vi "SCE_screen_main.vi"() -> ()   [LabVIEW 2018]
uses:
  SCE_VIC-II_registry.ctl
  SCE_character_bitmap.ctl
  CIA/CIA1/CIA1_glb.vi
panel:
  out "matrix":bool[][](array[boolean])
  out "VIC-II":T1
  out "Charset ROM":path=path "D:/work/experimets/C64/rom/characters.901225-01.bin"
  out "main time":u32
  out "Current State":string
  out "screen":picture
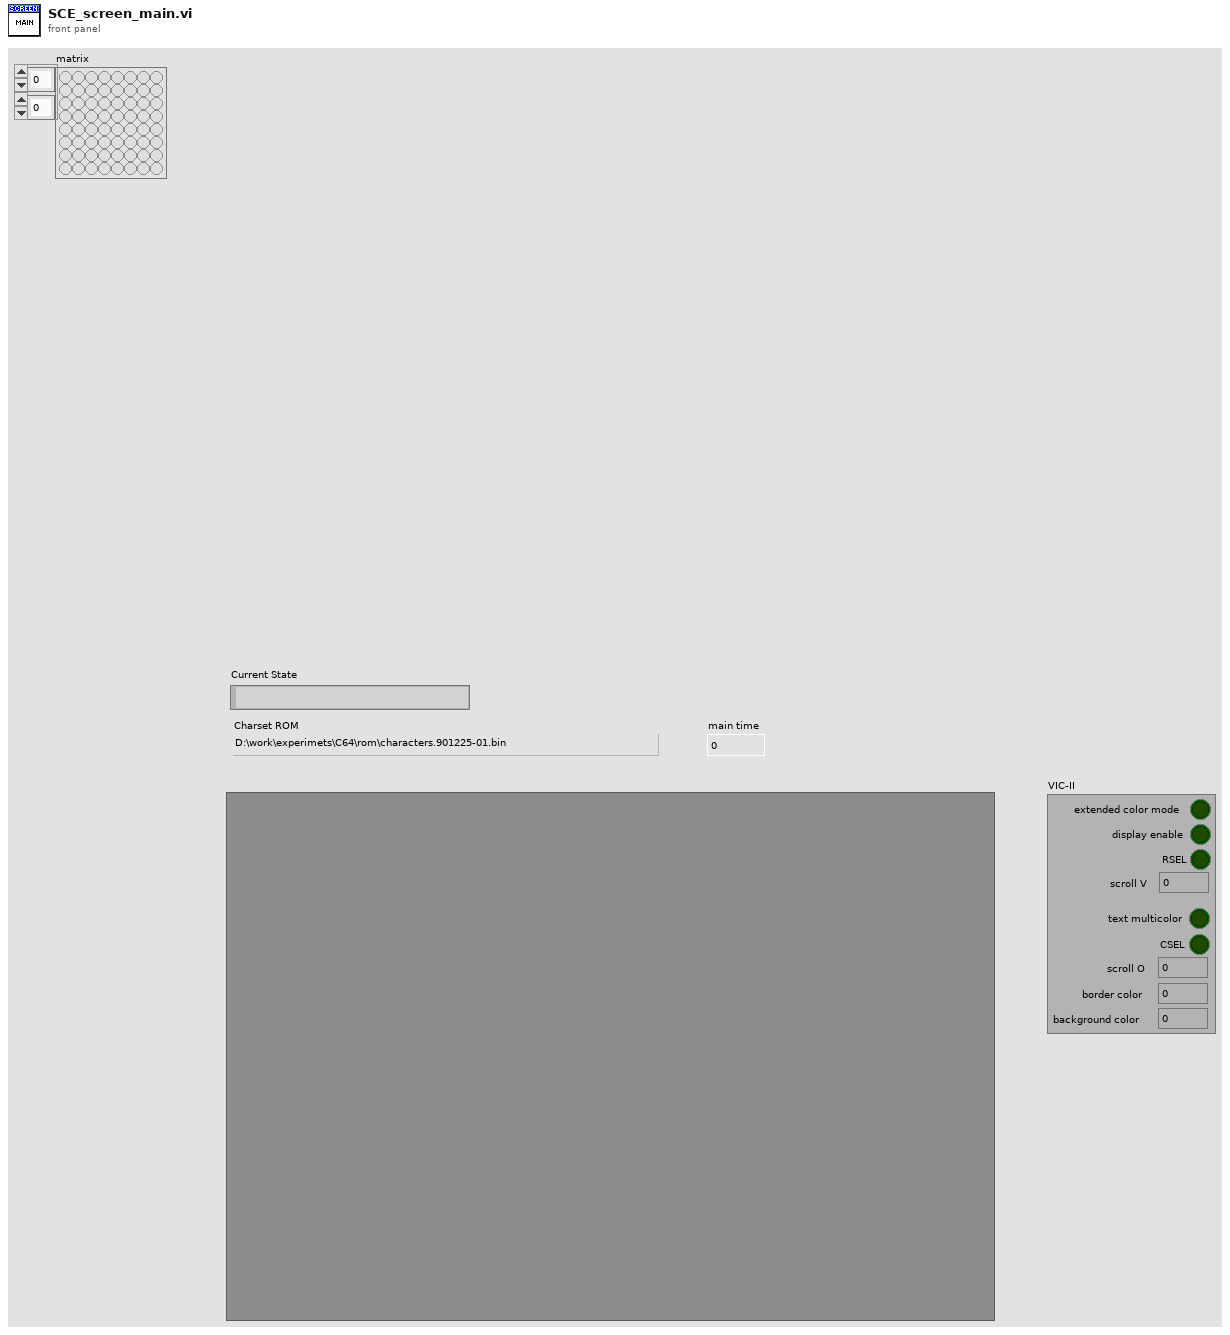
[diagram p1: front panel]
types:
  T1 = typedef "SCE_VIC-II_registry.ctl" = cluster{"extended color mode":bool, "display enable":bool, "RSEL":bool, "scroll V":u8, "text multicolor":bool, "CSEL":bool, "scroll O":u8, "border color":u8, "background color":u8}
  T2 = typedef "SCE_character_bitmap.ctl" = cluster{"ID":i32, "character bitmap":u8[][]}
  T3 = typedef "SCE_VIC-II_reg_D018.ctl" = cluster{"charset mode":enum16{"ROM set 1", "ROM set 2", "RAM"}, "charset addr":u16, "video ram addr":u16}
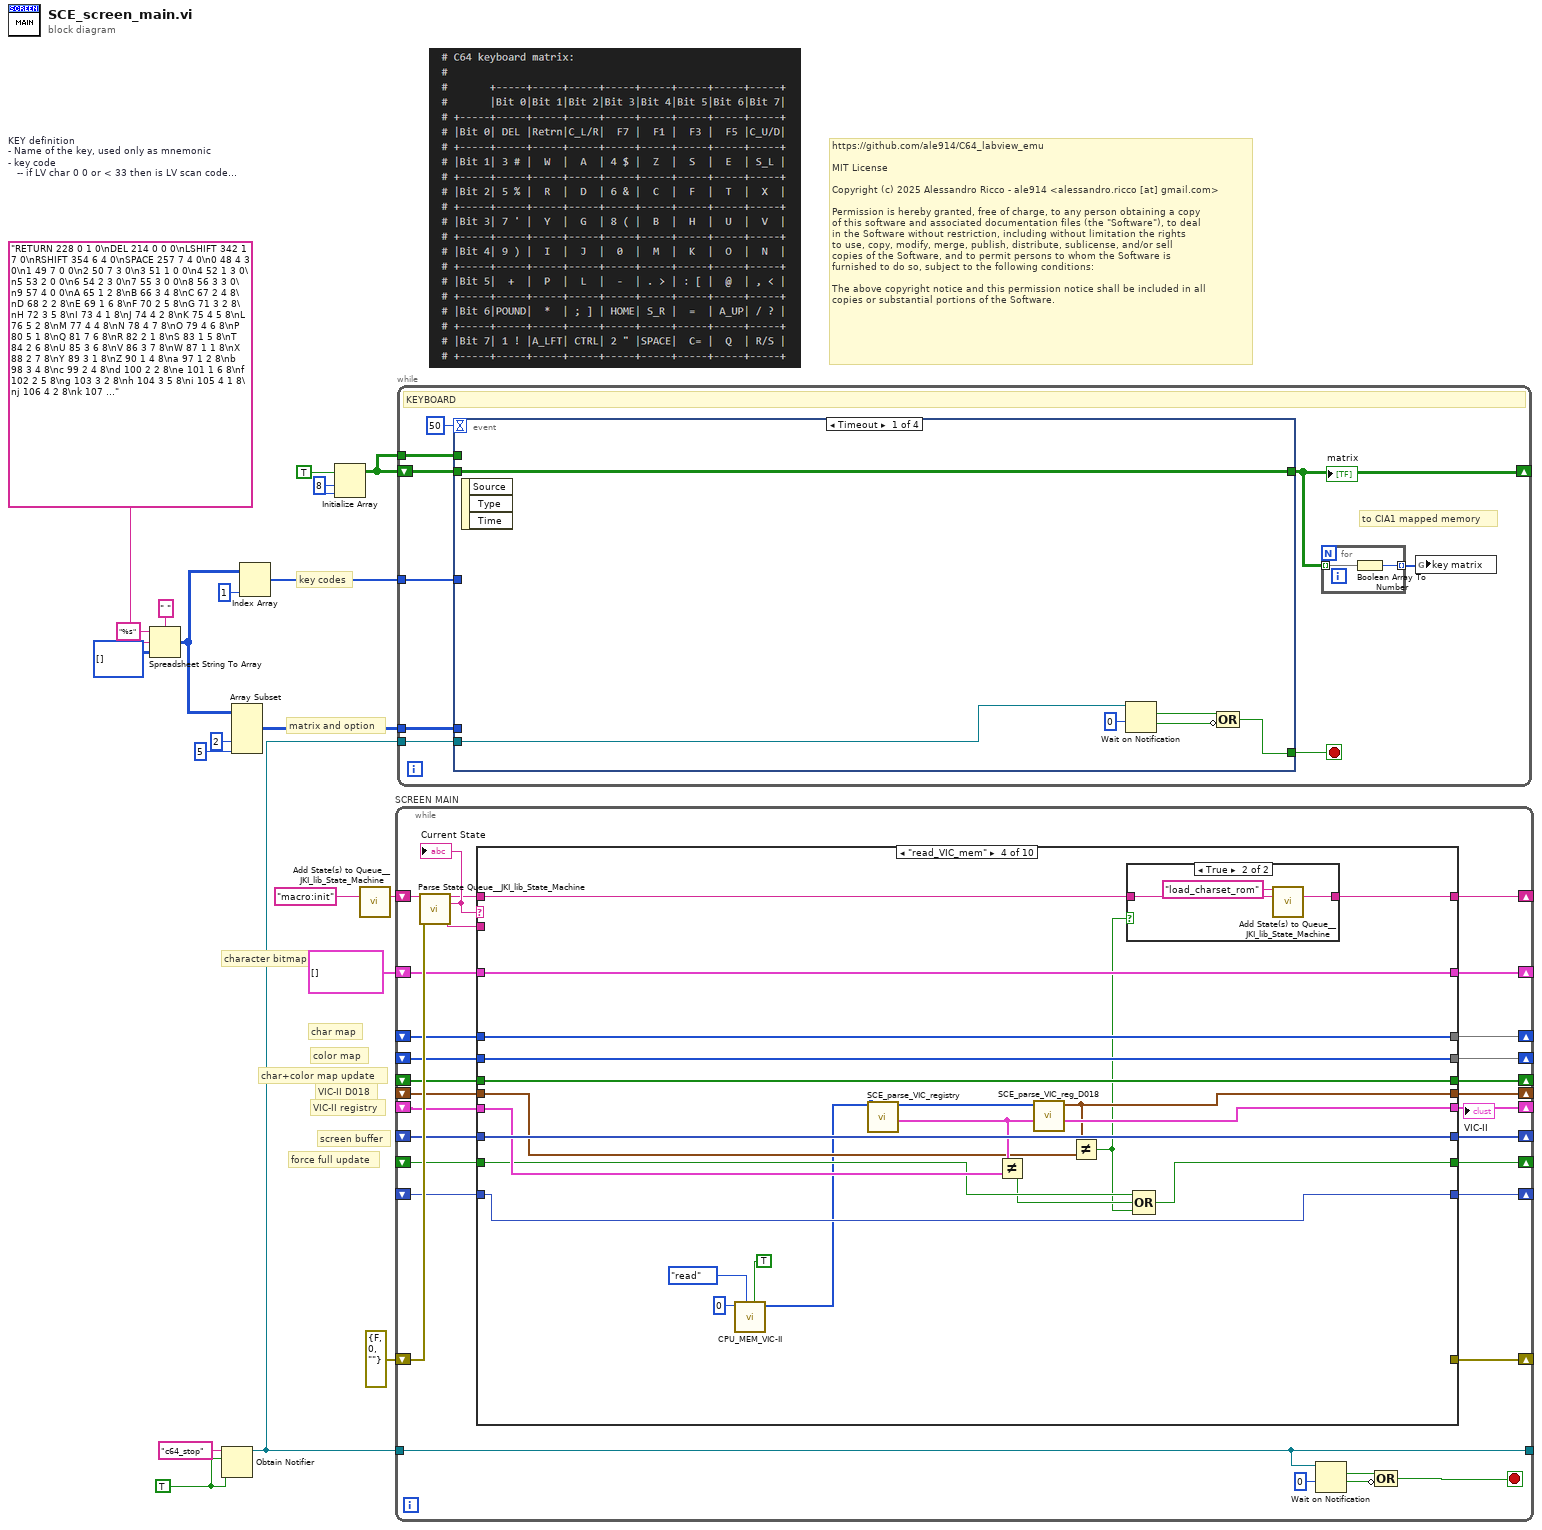
[diagram p0: block diagram]
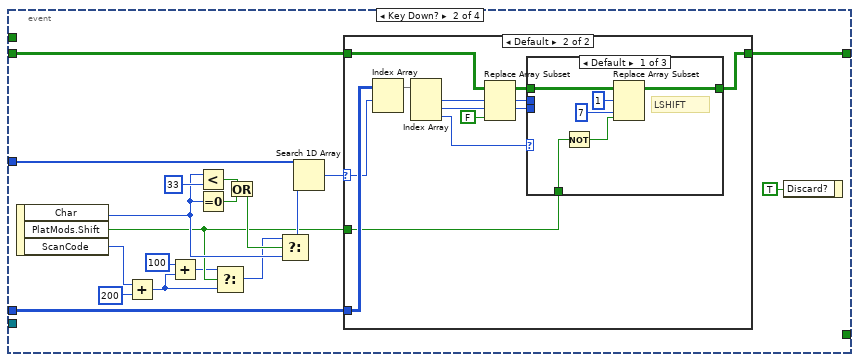
[diagram p2: hidden frame]
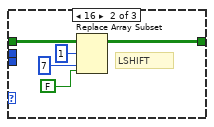
[diagram p4: hidden frame]
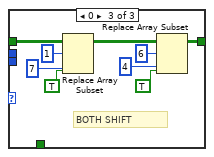
[diagram p5: hidden frame]
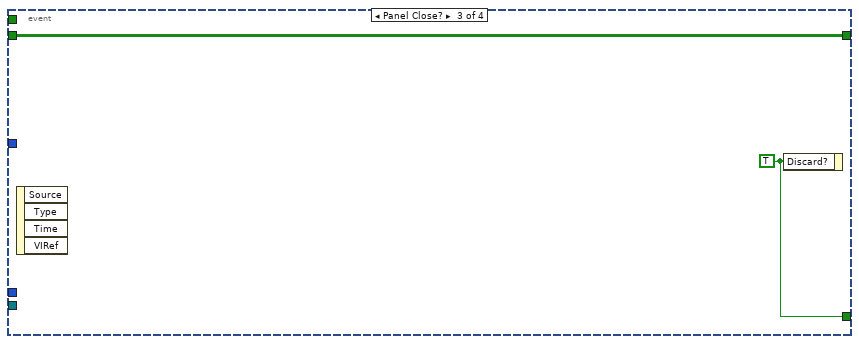
[diagram p6: hidden frame]
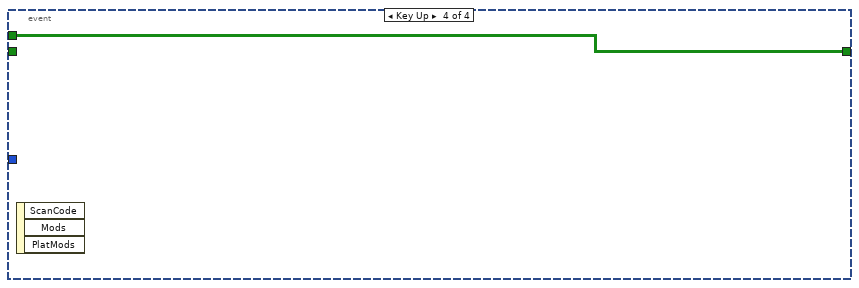
[diagram p7: hidden frame]
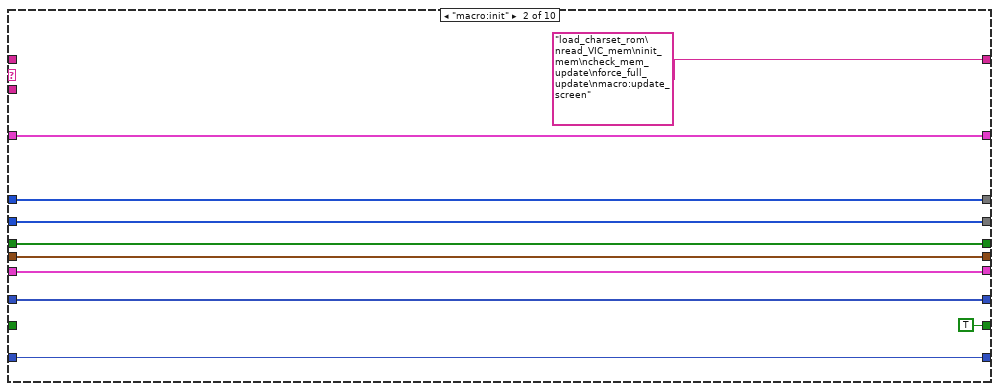
[diagram p9: hidden frame]
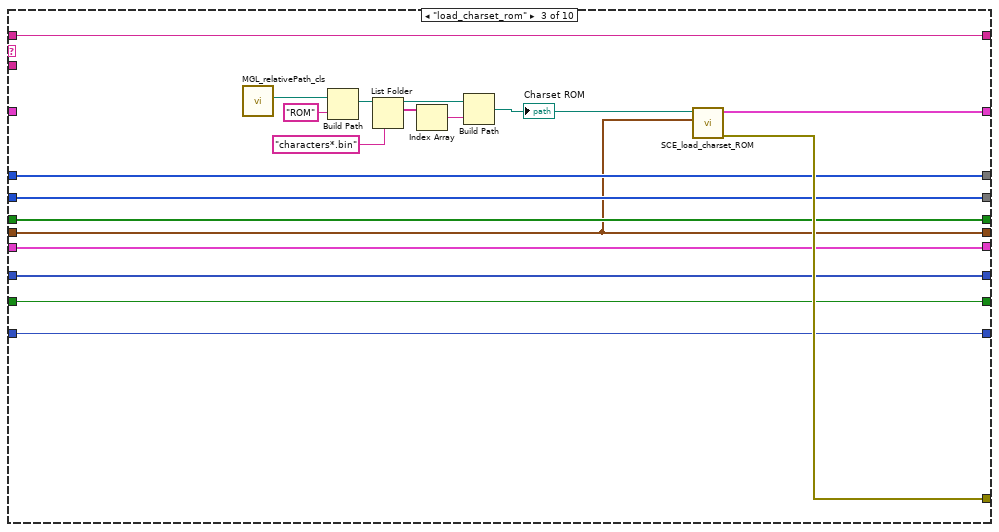
[diagram p10: hidden frame]
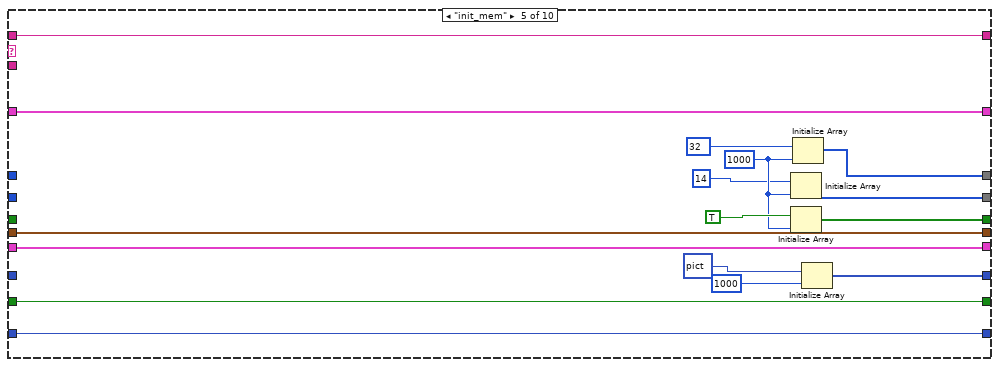
[diagram p12: hidden frame]
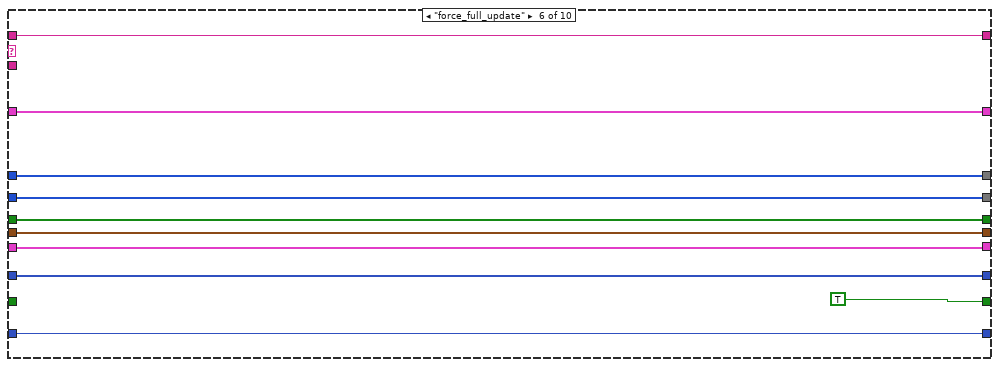
[diagram p13: hidden frame]
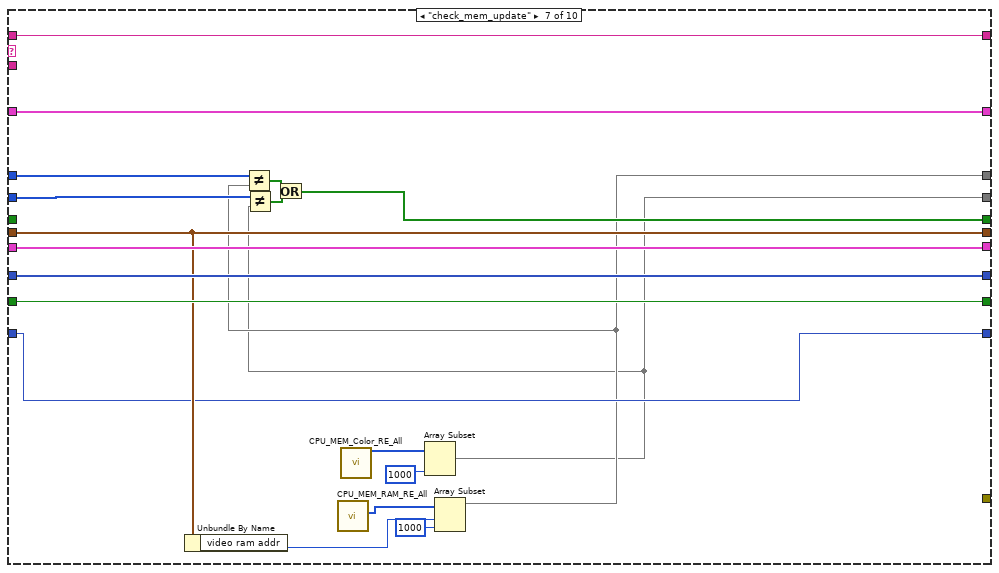
[diagram p14: hidden frame]
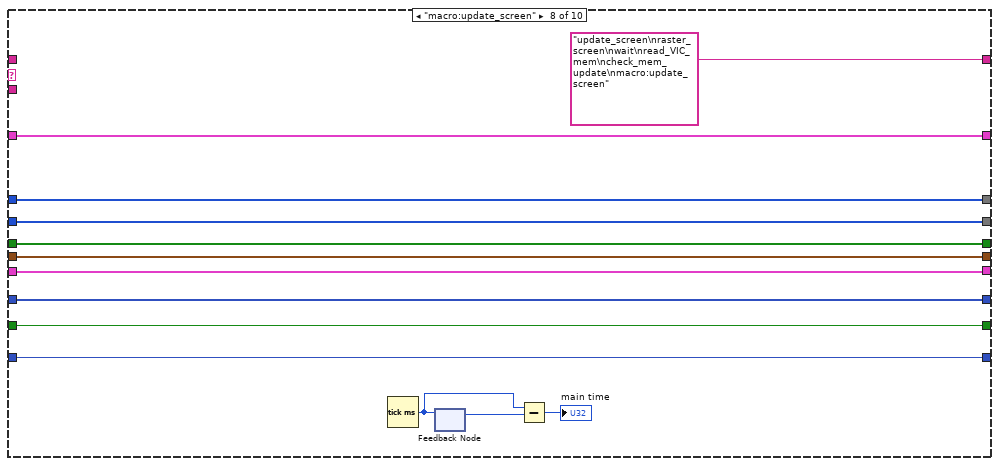
[diagram p15: hidden frame]
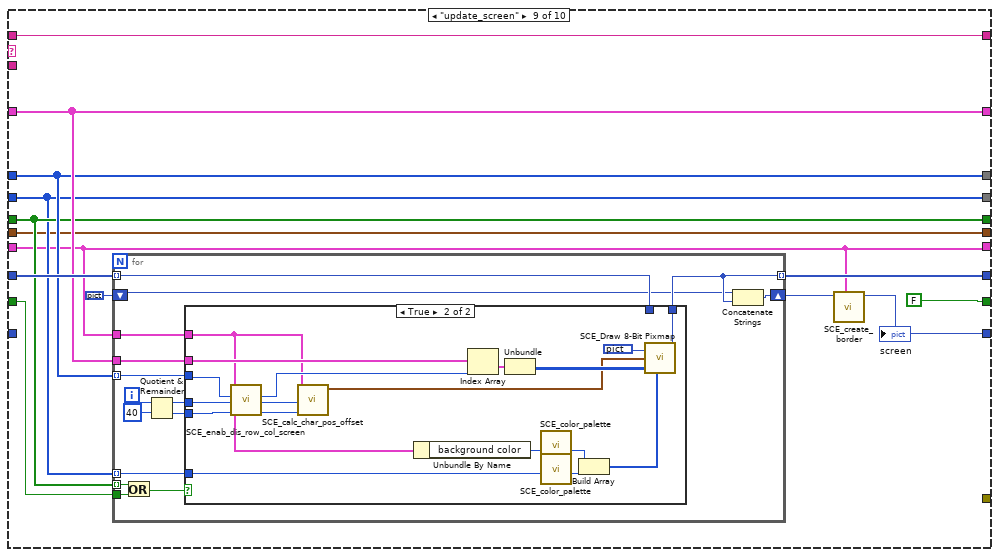
[diagram p16: hidden frame]
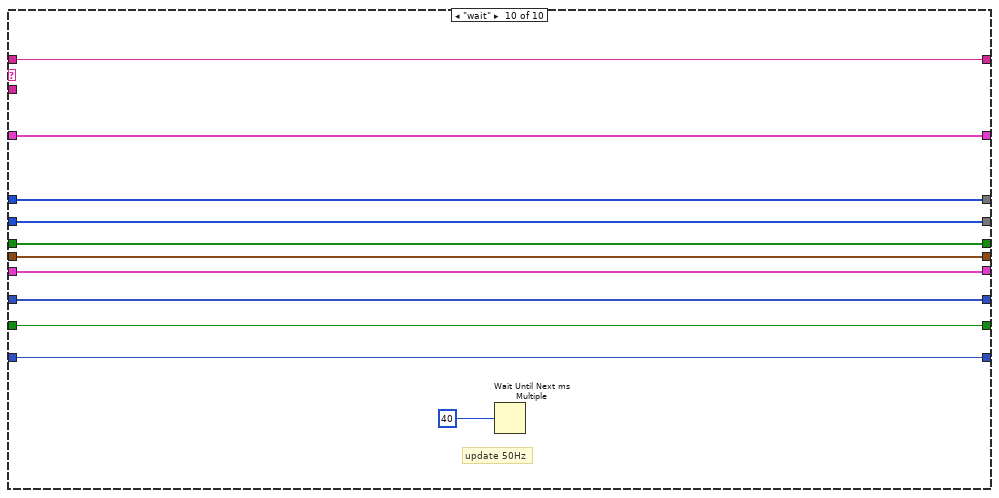
[diagram p18: hidden frame]
diagram:
  w12 = "RETURN 228 0 1 0\nDEL 214 0 0 0\nLSHIFT 342 1 7 0\nRSHIFT 354 6 4 0\nSPACE 257 7 4 0\n0 48 4 3 0\n1 49 7 0 0\n2 50 7 3 0\n3 51 1 0 0\n4 52 1 3 0\n5 53 2 0 0\n6 54 2 3 0\n7 55 3 0 0\n8 56 3 3 0\n9 57 4 0 0\nA 65 1 2 8\nB 66 3 4 8\nC 67 2 4 8\nD 68 2 2 8\nE 69 1 6 8\nF 70 2 5 8\nG 71 3 2 8\nH 72 3 5 8\nI 73 4 1 8\nJ 74 4 2 8\nK 75 4 5 8\nL 76 5 2 8\nM 77 4 4 8\nN 78 4 7 8\nO 79 4 6 8\nP 80 5 1 8\nQ 81 7 6 8\nR 82 2 1 8\nS 83 1 5 8\nT 84 2 6 8\nU 85 3 6 8\nV 86 3 7 8\nW 87 1 1 8\nX 88 2 7 8\nY 89 3 1 8\nZ 90 1 4 8\na 97 1 2 8\nb 98 3 4 8\nc 99 2 4 8\nd 100 2 2 8\ne 101 1 6 8\nf 102 2 5 8\ng 103 3 2 8\nh 104 3 5 8\ni 105 4 1 8\nj 106 4 2 8\nk 107 4 5 8\nl 108 5 2 8\nm 109 4 4 8\nn 110 4 7 8\no 111 4 6 8\np 112 5 1 8\nq 113 7 6 8\nr 114 2 1 8\ns 115 1 5 8\nt 116 2 6 8\nu 117 3 6 8\nv 118 3 7 8\nw 119 1 1 8\nx 120 2 7 8\ny 121 3 1 8\nz 122 1 4 8\n? 63 6 7 16\n/ 47 6 7 0\n# 35 1 0 16\n$ 36 1 3 16\n% 37 2 0 16\n& 38 2 3 16\n' 39 3 0 16\n( 40 3 3 16\n) 41 4 0 16\n+ 43 5 0 0\n- 45 5 3 0\n- 46 5 4 0\n> 62 5 4 16\n: 58 5 5 0\n[ 91 5 5 16\n@ 64 5 6 0\n, 44 5 7 0\n< 60 5 7 16\n£ 163 6 0 0\n* 42 6 1 0\n; 59 6 2 0\n] 93 6 2 16\n= 61 6 5 0\n! 33 7 0 16\nCTRL 229 7 2 0\n\" 34 7 3 16\nC64 215 7 5 0\nC64_S 315 7 5 16\nARR_LEFT 375 7 1 0\nARR_UP 372 6 6 0\nCUR_LEFT 277 0 2 0\nCUR_RIGTH 275 0 2 16\nCUR_UP 280 0 7 0\nCUR_UP 272 0 7 16\nRUN 201 7 7 0\nF7 265 0 3 0\nF1 259 0 4 0\nF3 261 0 5 0\nF5 263 0 6 0\n"  # KEY definition - Name of the key, used only as mnemonic - key code    -- if LV char 0 0 or < 33 then is LV scan code +200 or +300 if shift is pressed        otherwise is LV char directly - C64 matrix row - C64 matrix column - shift modifier,        --  0 = shift inhibit        -- 16 = shift forced        -- default = shift passed to c64 matrix as pressed
  w14 = 8 ("dimension size")
  w15 = TRUE ("create if not found? (T)")
  # "https://github.com/ale914/C64_labview_emu\n\nMIT License\n\nCopyright (c) 2025 Alessandro Ricco - ale914 <alessandro.ricco [at] gmail.com>\n\nPermission is hereby granted, free of charge, to any person obtaining a copy\nof this software and associated documentation files (the \"Software\"), to deal\nin the Software without restriction, including without limitation the rights\nto use, copy, modify, merge, publish, distribute, sublicense, and/or sell\ncopies of the Software, and to permit persons to whom the Software is\nfurnished to do so, subject to the following conditions:\n\nThe above copyright notice and this permission notice shall be included in all\ncopies or substantial portions of the Software."
  # "matrix and option"
  # "key codes"
  # "VIC-II D018"
  # "VIC-II registry"
  # "force full update"
  # "screen buffer"
  # "char+color map update"
  # "color map"
  # "char map"
  # "character bitmap"
  n1 = Spreadsheet String To Array(delimiter (Tab)=" ", format string="%s", spreadsheet string=w12, array type (2D Dbl)=i32[][] []) -> (array=w6:i32[][])
  n2 = Obtain Notifier(name (unnamed)="c64_stop", notification data type=w15, create if not found? (T)=w15) -> (notifier out=w1:refnum<notifier>)  [unwired: 1 in, 2 out]
  n3 = Array Subset(array=w6, index (col)=2 ("index"), length (col)=5 ("length")) -> (w2:i32[][])  [unwired: 2 in]
  n4 = Index Array(array=w6, index (col)=1 ("disabled index (col)")) -> (element=w7:i32[])  [unwired: 1 in]
  n5 = Initialize Array(TRUE, w14, w14) -> (w3:bool[][])
  n6 = call "Add State(s) to Queue__JKI_lib_State_Machine.vi"("State(s) in (\"\")"="macro:init") -> ("States Out"=w20:string)  [unwired: 14 in]
  n7 = while "SCREEN MAIN" {
    shift-right: [w44] -> _
    shift-left: errorcluster {"status"=FALSE, "code"=0, "source"=""} ("error out") -> [w49]
    shift-right: [w45] -> _
    shift-left: w20 -> [w50]
    shift-right: [w43] -> _
    shift-left: T2[] [] ("char set") -> [w42]
    shift-right: [w41] -> _
    shift-left: _ -> [w39]
    shift-right: [w40] -> _
    shift-left: _ -> [w38]
    shift-right: [w37] -> _
    shift-left: _ -> [w36]
    shift-right: [w35] -> _
    shift-left: _ -> [w34]
    shift-right: [w32] -> _
    shift-left: _ -> [w33]
    shift-right: [w31] -> _
    shift-left: _ -> [w30]
    shift-right: [w29] -> _
    shift-left: _ -> [w28]
    shift-right: [w27] -> _
    shift-left: _ -> [w26]
    tunnel: w1 -> [w22]
    tunnel: [w22] -> _
    stop <- w21 stop-if-true
    n8 = call "Parse State Queue__JKI_lib_State_Machine.vi"("State Queue"=w50, "Error In (no error)"=w49) -> ("Remaining States"=w47:string, "Current State"=w48:string, "Arguments"=w46:string)  [unwired: 11 in]
    "Current State" <- w48
    n9 = case shown="\"read_VIC_mem\"" w48 {
      tunnel: w47 -> [w54 _ w87 w96 w129 w139 w158 _ w185 w224]
      tunnel: w46 -> [_ _ _ _ _ _ _ _ _ _]
      tunnel: [w54 "load_charset_rom\nread_VIC_mem\ninit_mem\ncheck_mem_update\nforce_full_update\nmacro:update_screen" ("Remaining States") w87 w97 w129 w139 w158 "update_screen\nraster_screen\nwait\nread_VIC_mem\ncheck_mem_update\nmacro:update_screen" ("Remaining States") w185 w224] -> w45
      tunnel: [_ _ w88 _ _ _ _ _ _ _] -> w44
      tunnel: [w60 w69 w89 w109 w128 w138 w157 w170 w182 w228] -> w43
      tunnel: w42 -> [w60 w69 _ w109 w128 w138 w157 w170 w182 w228]
      tunnel: [w59 w68 w86 w108 w119 w136 w146 w169 w181 w227] -> w41
      tunnel: [w58 w67 w85 w107 w116 w137 w141 w168 w179 w226] -> w40
      tunnel: w39 -> [w59 w68 w86 w108 _ w136 w156 w169 w181 w227]
      tunnel: w38 -> [w58 w67 w85 w107 _ w137 w155 w168 w179 w226]
      tunnel: [w57 w66 w84 w106 w126 w134 w152 w167 w180 w225] -> w37
      tunnel: w36 -> [w57 w66 w84 w106 _ w134 _ w167 w180 w225]
      tunnel: [w56 w65 w83 w105 w121 w135 w151 w166 w183 w222] -> w35
      tunnel: w34 -> [w56 w65 w83 w105 _ w135 w151 w166 w184 w222]
      tunnel: w33 -> [w55 _ w82 w100 w124 _ w150 w165 w174 w221]
      tunnel: [w55 TRUE w82 w98 w124 TRUE w150 w165 FALSE w221] -> w32
      tunnel: [w53 w64 w81 w104 w120 w132 w149 w164 w176 w220] -> w31
      tunnel: w30 -> [w53 w64 w81 w103 w120 w132 w149 w164 w176 w220]
      tunnel: [w52 w63 w80 w102 w115 w131 w148 w163 w175 w219] -> w29
      tunnel: w28 -> [w52 w63 w80 w101 w115 w131 w148 w163 w175 w219]
      tunnel: [w51 w62 w79 w94 w114 w130 w147 w159 w172 w218] -> w27
      tunnel: w26 -> [w51 w62 w79 w94 w114 w130 w147 w159 _ w218]
      frame "idle", Default {
      }
      frame "macro:init" {
      }
      frame "load_charset_rom" {
        n10 = call "MGL_relativePath_cls.vi"() -> ("Path"=w78:path)  [unwired: 8 in, 1 out]
        n11 = Build Path(base path=w78, name or relative path="ROM") -> (appended path=w75:path)
        n12 = List Folder(path=w75, pattern="characters*.bin") -> (path out=w73:path, filenames=w74:string[])  [unwired: 2 in, 2 out]
        n13 = Index Array(array=w74) -> (element=w72:string)  [unwired: 1 in]
        n14 = Build Path(base path=w73, name or relative path=w72) -> (appended path=w71:path)
        "Charset ROM" <- w71
        n15 = call "SCE_load_charset_ROM.vi"("VIC-II D018"=w80, "Charset ROM"=w71) -> ("error out"=w88:errorcluster, "char set"=w89:T2[])  [unwired: 8 in]
      }
      frame "read_VIC_mem" {
        n16 = call "CPU_MEM_VIC-II.vi"("read all"=TRUE, "oper"=enum16{"init", "read", "write"}."read", "address"=u16 0) -> ("mem"=w90:u8[])  [unwired: 7 in, 1 out]
        n17 = call "SCE_parse_VIC_registry.vi"("$D000 - $D03F"=w90) -> ("VIC-II"=w104:T1)  [unwired: 10 in]
        n18 = Not Equal?(x=w104, y=w103) -> (x != y?=w99:bool)
        n19 = call "SCE_parse_VIC_reg_D018.vi"("$D000 - $D03F"=w90) -> ("VIC-II D018"=w102:T3)  [unwired: 10 in]
        n20 = Not Equal?(x=w102, y=w101) -> (x != y?=w95:bool)
        n21 = case shown="True" w95 {
          tunnel: [w110 w113] -> w97
          tunnel: w96 -> [w110 w112]
          frame False {
          }
          frame True {
            n22 = call "Add State(s) to Queue__JKI_lib_State_Machine.vi"("State(s) in Front (\"\")"="load_charset_rom" ("State(s) in Front (\"\")"), "State(s) in (\"\")"=w112) -> ("States Out"=w113:string)  [unwired: 13 in]
          }
        }
        n23 = Compound Arithmetic op=OR(w100, w99, w95) -> (w98:bool)
      }
      frame "init_mem" {
        w118 = 1000 ("dimension size")
        n24 = Initialize Array(u8 14 ("dimension size"), w118) -> (w116:u8[])
        n25 = Initialize Array(TRUE, w118) -> (w126:bool[])
        n26 = Initialize Array(u8 32 ("dimension size"), w118) -> (w119:u8[])
        n27 = Initialize Array(picture data[5B] ("new picture"), 1000 ("dimension size")) -> (w121:picture[])
      }
      frame "force_full_update" {
      }
      frame "check_mem_update" {
        n28 = Unbundle By Name(w148) -> ("video ram addr"=w143:u16)
        n29 = call "CPU_MEM_RAM_RE_All.vi"() -> ("mem"=w144:u8[])  [unwired: 11 in]
        n30 = call "CPU_MEM_Color_RE_All.vi"() -> ("mem"=w142:u8[])  [unwired: 11 in]
        n31 = Array Subset(array=w142, length=1000) -> (w141:u8[])  [unwired: 1 in]
        n32 = Not Equal?(x=w155, y=w141) -> (x != y?=w153:bool[])
        n33 = Array Subset(array=w144, index=w143, length=1000) -> (w146:u8[])
        n34 = Not Equal?(x=w156, y=w146) -> (x != y?=w154:bool[])
        n35 = Or(x=w154, y=w153) -> (x .or. y?=w152:bool[])
      }
      frame "macro:update_screen" {
        n36 = Tick Count (ms)() -> (millisecond timer value=w161:u32)
        n37 = feedback-in #1(w161) -> ()
        n38 = feedback #1() -> (w162:u32)  [unwired: 1 in]
        n39 = Subtract(x=w161, y=w162) -> (x-y=→"main time":u32)
      }
      frame "update_screen" {
        n40 = for {
          tunnel: w182 -> [w200]
          tunnel: w181 -> [w199] mode=indexing
          tunnel: [w198] -> w183 mode=indexing
          shift-right: [w195] -> w173
          shift-left: picture data[5B] ("picture") -> [w196]
          tunnel: w184 -> [w197] mode=indexing
          tunnel: w179 -> [w194] mode=indexing
          tunnel: w180 -> [w188] mode=indexing
          tunnel: w174 -> [w187]
          tunnel: w176 -> [w186]
          i -> [w191]
          n41 = Or(x=w188, y=w187) -> (x .or. y?=w189:bool)
          n42 = Quotient & Remainder(x=w191, y=40) -> (x-y*floor(x/y)=w192:i32, floor(x/y)=w190:i32)
          n43 = case shown="True" w189 {
            tunnel: w200 -> [_ w217]
            tunnel: w199 -> [_ w211]
            tunnel: [w201 w213] -> w198
            tunnel: w197 -> [w201 _]
            tunnel: w194 -> [_ w207]
            tunnel: w192 -> [_ w210]
            tunnel: w190 -> [_ w209]
            tunnel: w186 -> [_ w205]
            frame False {
            }
            frame True {
              n44 = call "SCE_enab_dis_row_col_screen.vi"("row"=w209, "col"=w210, "char ID"=w211, "VIC-II"=w205) -> ("char ID out"=w212:i32)  [unwired: 7 in]
              n45 = call "SCE_calc_char_pos_offset.vi"("row"=w209, "col"=w210, "VIC-II"=w205) -> ("pos"=w208:cluster{"x":i16, "y":i16})  [unwired: 8 in]
              n46 = Unbundle By Name(w205) -> ("background color"=w204:u8)
              n47 = Index Array(array=w217, index=w212) -> (element=w216:T2)
              n48 = Unbundle(w216) -> ("character bitmap"=w215:u8[][])  [unwired: 1 out]
              n49 = call "SCE_color_palette.vi"("color index"=w204) -> ("selected color"=w203:u32)  [unwired: 9 in, 1 out]
              n50 = call "SCE_color_palette.vi"("color index"=w207) -> ("selected color"=w206:u32)  [unwired: 9 in, 1 out]
              n51 = Build Array(w203, w206) -> (w202:u32[])
              n52 = call "SCE_Draw 8-Bit Pixmap.vi"("picture"=picture data[5B], "top left point(0, 0)"=w208, "data"=w215, "color table"=w202) -> ("new picture"=w213:picture)  [unwired: 5 in]
            }
          }
          n53 = Concatenate Strings(w196, w198) -> (w195:picture)
        }
        n54 = call "SCE_create_border.vi"("VIC-II"=w176, "screen in"=w173) -> ("screen out"=w172:picture)  [unwired: 9 in]
        "screen" <- w172
      }
      frame "wait" {
        # "update 50Hz"
        n55 = Wait Until Next ms Multiple(millisecond multiple=u32 40 ("milliseconds to wait")) -> ()  [unwired: 1 out]
      }
    }
    "VIC-II" <- w31
    n56 = Wait on Notification(notifier=w22, timeout in ms (-1)=0) -> (notification=w24:bool, timed out?=w23:bool)  [unwired: 2 in, 2 out]
    n57 = Compound Arithmetic op=OR(w24, invert w23) -> (w21:bool)
  }
  n58 = while {
    shift-right: [w232] -> _
    shift-left: w3 -> [w237]
    tunnel: w7 -> [w235]
    tunnel: w2 -> [w234]
    tunnel: w3 -> [w231]
    tunnel: w1 -> [w229]
    stop <- w230 stop-if-true
    # "to CIA1 mapped memory"
    # "KEYBOARD"
    n59 = event shown="[0] Timeout" {
      selector: _ -> [_ _ _ _]
      dyn-events: _ -> [_ _ _ _]
      timeout: 50 -> [_ _ _ _]
      tunnel: w237 -> [w245 w261 w297 _]
      tunnel: w235 -> [_ w263 _ _]
      tunnel: [w245 w260 w297 w299] -> w232
      tunnel: w234 -> [_ w259 _ _]
      tunnel: w231 -> [_ _ _ w299]
      tunnel: [w240 _ w298 _] -> w230
      tunnel: w229 -> [w243 _ _ _]
      event Timeout {
        n60 = event-data() -> ()  [unwired: 1 in, 3 out]
        n61 = Wait on Notification(notifier=w243, timeout in ms (-1)=0) -> (notification=w242:bool, timed out?=w241:bool)  [unwired: 2 in, 2 out]
        n62 = Compound Arithmetic op=OR(w242, invert w241) -> (w240:bool)
      }
      event Key Down? {
        n63 = event-data() -> ("Char"=w255:i16, "PlatMods.Shift"=w250:bool, "ScanCode"=w251:i16)  [unwired: 1 in]
        n64 = Add(x=w251, y=i16 200) -> (x+y=w248:i16)
        n65 = Add(x=i16 100 ("y"), y=w248) -> (x+y=w249:i16)
        n66 = Less?(x=w255, y=i16 33) -> (x < y?=w258:bool)
        n67 = Equal To 0?(x=w255) -> (x = 0?=w253:bool)
        n68 = Select(t=w249, s=w250, f=w248) -> (s? t:f=w247:i16)
        n69 = Or(x=w258, y=w253) -> (x .or. y?=w254:bool)
        n70 = Select(t=w247, s=w254, f=w255) -> (s? t:f=w256:i16)
        n71 = Search 1D Array(1D array=w263, element=w256) -> (index of element=w262:i32)  [unwired: 1 in]
        n72 = case shown="Default" w262 {
          selector: w262 -> [_ w272]
          tunnel: w261 -> [w265 w275]
          tunnel: [w265 w269] -> w260
          tunnel: w259 -> [_ w276]
          tunnel: w250 -> [_ w266]
          frame -1 {
          }
          frame Default {
            n73 = Index Array(array=w276, index (row)=w272) -> (element=w274:i32[])  [unwired: 1 in]
            n74 = Index Array(array=w274) -> (element #1=w268:i32, element #2=w267:i32, element #3=w271:i32)  [unwired: 3 in]
            n75 = Replace Array Subset(array=w275, new element=FALSE ("new element/subarray"), index (row)=w268, index (col)=w267) -> (w270:bool[][])
            n76 = case shown="Default" w271 {
              tunnel: w270 -> [w277 w287 w296]
              tunnel: [w278 w285 w288] -> w269
              tunnel: w268 -> [_ _ _]
              tunnel: w267 -> [_ _ _]
              tunnel: w266 -> [w280 _ _]
              frame Default {
                # "LSHIFT"
                n77 = Not(x=w280) -> (.not. x?=w279:bool)
                n78 = Replace Array Subset(array=w277, new element=w279, index (row)=1, index (col)=7 ("disabled index (col)")) -> (w278:bool[][])
              }
              frame 16 {
                # "LSHIFT"
                n79 = Replace Array Subset(array=w287, new element=FALSE, index (row)=1, index (col)=7 ("disabled index (col)")) -> (w285:bool[][])
              }
              frame 0 {
                # "BOTH SHIFT"
                n80 = Replace Array Subset(array=w296, new element=TRUE, index (row)=1, index (col)=7 ("disabled index (col)")) -> (w289:bool[][])
                n81 = Replace Array Subset(array=w289, new element=TRUE, index (row)=6, index (col)=4 ("disabled index (col)")) -> (w288:bool[][])
              }
            }
          }
        }
        n82 = event-data("Discard?"=TRUE) -> ()  [unwired: 1 in, 1 out]
      }
      event Panel Close? {
        w298 = TRUE ("Discard?")
        n83 = event-data() -> ()  [unwired: 1 in, 4 out]
        n84 = event-data("Discard?"=w298) -> ()  [unwired: 1 in, 1 out]
      }
      event Key Up {
        n85 = event-data() -> ()  [unwired: 1 in, 3 out]
      }
    }
    "matrix" <- w232
    n86 = for {
      tunnel: w232 -> [w238] mode=indexing
      tunnel: [w239] -> w233 mode=indexing
      n87 = Boolean Array To Number(Boolean array=w238) -> (number=w239:u8)
    }
    n88 = global write "CIA1_glb.vi" "key matrix"(w233) -> ()
  }
